vi "absolute_link_PTH.vi"() -> ()   [LabVIEW 2021]
panel:
  in  "PTH":path
  # "PTH"
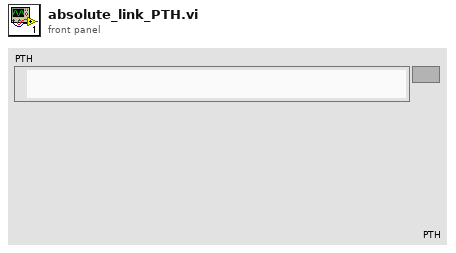
[diagram p1: front panel]
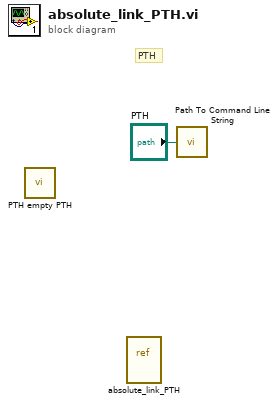
[diagram p0: block diagram]
diagram:
  # "PTH"
  n1 = call "PTH empty PTH.vi"() -> ()  [unwired: 12 in]
  n2 = vi-ref "absolute_link_PTH.vi"() -> ()  [unwired: 1 out]
  n3 = call <vilib>:"Path To Command Line String.vi"("path"="PTH") -> ()  [unwired: 1 out]
